vi "Remove Empty Keys.vi"(11 "keyed array":T1) -> (3 "keyed array":T1)   [LabVIEW 2012, in "TLB` Template.lvlib" / "Tools_KeyedArray.lvlib"]
uses:
  Tools_KeyedArray.lvlib
  KeyedArray.ctl
  Map String.vi
  String/Get Case Matching.vi
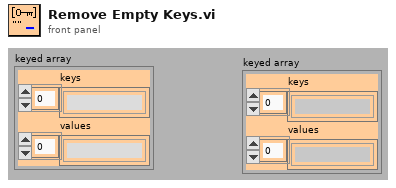
[diagram p1: front panel]
types:
  T1 = typedef "TLB` Template.lvlib/Tools_KeyedArray.lvlib/KeyedArray.ctl" = cluster{"keys":string[], "values":string[]}
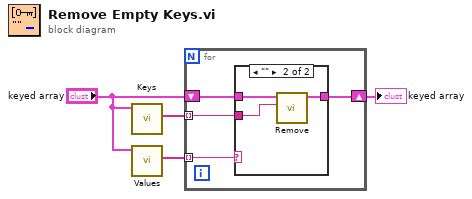
[diagram p0: block diagram]
diagram:
  n1 = call "Keys.vi"("array in"="keyed array") -> ("keys"=w2:string[])  [unwired: 6 out]
  n2 = call "Values.vi"("array in"="keyed array") -> ("values"=w3:string[])  [unwired: 6 out]
  n3 = for {
    shift-right: [w7] -> w1
    shift-left: "keyed array" -> [w8]
    tunnel: w3 -> [w6] mode=indexing
    tunnel: w2 -> [w5] mode=indexing
    n4 = case shown="\"\"" w6 {
      tunnel: [w9 w10] -> w7
      tunnel: w8 -> [w9 w12]
      tunnel: w5 -> [_ w11]
      frame Default {
      }
      frame "" {
        n5 = call "Remove.vi"("key"=w11, "array in"=w12) -> ("array out"=w10:T1)  [unwired: 1 in, 4 out]
      }
    }
  }
  "keyed array" <- w1
